vi "XIPIN_Image_Characterization_3_00_a.vi"   [LabVIEW 2017]
doc: "The Xilinx Image Characterization LogiCORE calculates important statistical data for video input streams. Characterization is an important processing block for many applications including face recognition, object detection, and more. Statistics include means and variances for luminance, chrominance, high and low frequencies, edges and motion (When used with the Xilinx Motion Adaptive Noise Reduction LogiCORE) on both a global and block basis. Support for block sizes of 4x4, 8x8, 16x16, 32x32 or 64x64 pixels. Support for 8-bit pixel data in YUV 4:2:2 or 4:2:0.\n------------------------------------\n<b>Need License</b> : Yes\n<b>Interface</b> : AXI4-Stream AXI4-Lite"
uses:
  <vilib>/rvi/XilinxIP/XIPIN_XNode/niFpgaXIPIN.xnode
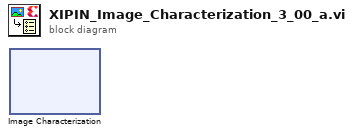
[diagram p0: block diagram]
diagram:
  n1 = xnode ("Image Characterization")() -> ()
